vi "encode fixed64.vi"(11 "U64":u64) -> (3 "byte array out":u8[](array[numeric]))   [LabVIEW 2013, in "protocol buffers encoder.lvlib"]
uses:
  protocol buffers encoder.lvlib
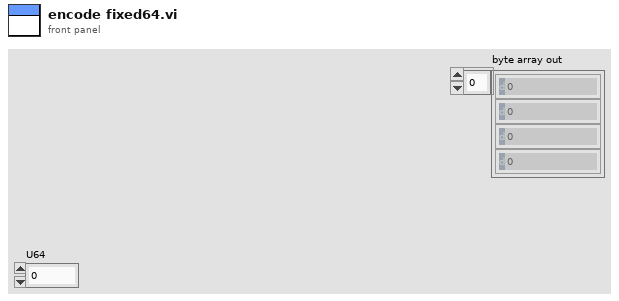
[diagram p1: front panel]
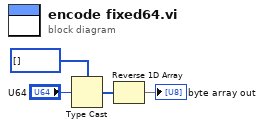
[diagram p0: block diagram]
diagram:
  n1 = Type Cast(type=u8[] [] ("byte array in"), x="U64") -> (*(type *) &x=w3:u8[])
  n2 = Reverse 1D Array(array=w3) -> (reversed array=→"byte array out":u8[])
